vi "Delete.vi"(8 "error in (no error)":errorcluster, 11 "Remote in":refnum<class "Remote.lvclass">) -> (0 "error out":errorcluster, 3 "Remote out":refnum<class "Remote.lvclass">)   [LabVIEW 2019, in "Remote.lvclass"]
uses:
  Remote.lvclass
  MatchData/MatchData.lvclass
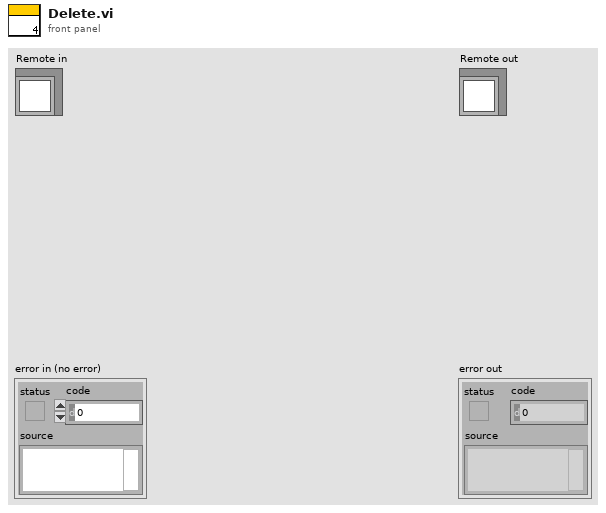
[diagram p1: front panel]
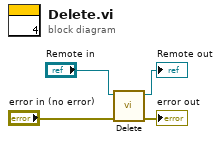
[diagram p0: block diagram]
diagram:
  n1 = call-parent "Delete.vi"("error in (no error)"="error in (no error)", "MatchData in"="Remote in") -> ("error out"=→"error out":errorcluster, "MatchData out"=→"Remote out":refnum<class "Remote.lvclass">)  [unwired: 8 in]
